vi "Error-example public API.vi"(8 "error to send":errorcluster, 11 "error in":errorcluster) -> (0 "error out":errorcluster)   [LabVIEW 2018]
doc: "Public API - enqueues error to queue of module."
uses:
  module/ctl/Module State--enum.ctl
  module/Template.lvlib
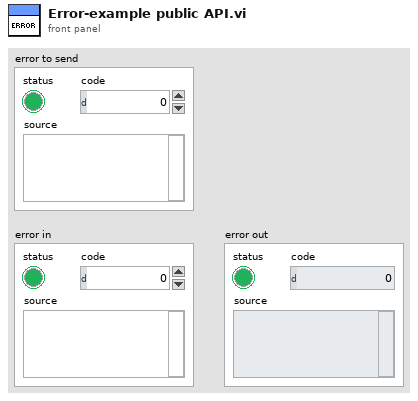
[diagram p1: front panel]
types:
  T1 = typedef "Template.lvlib/Module State--enum.ctl" = enum16{"Init", "Error", "Idle", "Close"}
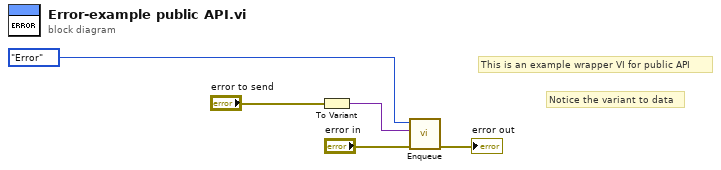
[diagram p0: block diagram]
diagram:
  # "Notice the variant to data"
  # "This is an example wrapper VI for public API"
  n1 = To Variant(anything="error to send") -> (Variant=w5:variant)
  n2 = call "Enqueue.vi"("error in (no error)"="error in", "Data"=w5, "State"=Module_State--enum."Error") -> ("error out"=→"error out":errorcluster)  [unwired: 8 in]
